vi "Get Function Type.vi"(8 "error in (no error)":errorcluster, 11 "VISA resource name":refnum<visa-resource-name>) -> (0 "error out":errorcluster, 2 "Function Type":i32, 3 "VISA resource name out":refnum<visa-resource-name>)   [LabVIEW 2013, in "Fluke 5XXX Series Multicalibrators.lvlib"]
doc: "This VI returns the present output, measurement, or calibration function.\n\nNote:\n\nThis VI is available only for instrument models 5500A and 5520A."
uses:
  Fluke 5XXX Series Multicalibrators.lvlib
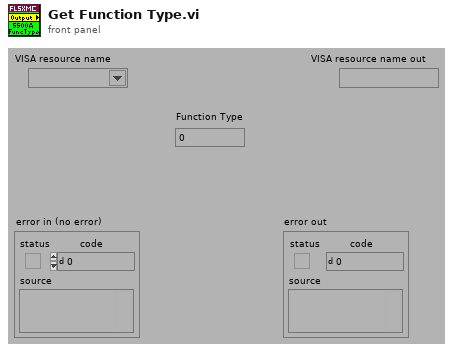
[diagram p1: front panel]
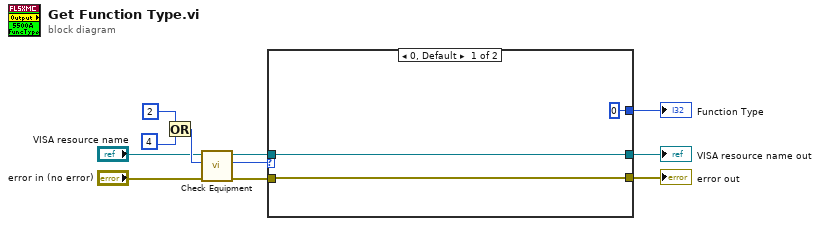
[diagram p0: block diagram]
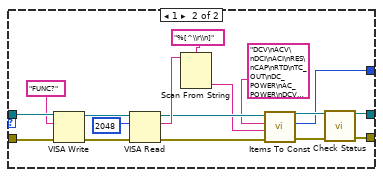
[diagram p2: hidden frame]
diagram:
  n1 = Or(x=2 ("Numeric"), y=4 ("Numeric")) -> (x .or. y?=w8:i32)
  n2 = call "Check Equipment.vi"("error in (no error)"="error in (no error)", "Bit Mask"=w8, "VISA resource name"="VISA resource name") -> ("error out"=w11:errorcluster, "Present?"=w10:u32, "VISA resource name out"=w9:refnum<visa-resource-name>)  [unwired: 6 in]
  n3 = case shown="0, Default" w10 {
    tunnel: [w13 w22] -> w2
    tunnel: w11 -> [w14 w30]
    tunnel: w9 -> [w13 w29]
    tunnel: [w14 w31] -> w3
    tunnel: [0 ("Index") w16] -> w1
    frame 0, Default {
    }
    frame 1 {
      n4 = VISA Write(VISA resource name=w29, write buffer="FUNC?", error in (no error)=w30) -> (VISA resource name out=w26:refnum<visa-resource-name>, error out=w25:errorcluster)  [unwired: 1 out]
      n5 = VISA Read(VISA resource name=w26, byte count=u32 2048 ("byte count (0)"), error in (no error)=w25) -> (VISA resource name out=w19:refnum<visa-resource-name>, read buffer=w23:string, error out=w18:errorcluster)  [unwired: 1 out]
      n6 = Scan From String(format string="%[^\\r\\n]", input string=w23) -> (output 1=w17:string)  [unwired: 3 in, 3 out]
      n7 = call "Items To Const.vi"("error in (no error)"=w18, "String Item"=w17, "Multi-Line String"="DCV\nACV\nDCI\nACI\nRES\nCAP\nRTD\nTC_OUT\nDC_POWER\nAC_POWER\nDCV_DCV\nACV_ACV\nTC_MEAS\nSACV\nSDCV\nMARKER\nLEVSINE\nEDGE\nWAVEGEN\nVIDEO\nPULSE\nMEASZ\nOVERLD", "VISA resource name"=w19) -> ("error out"=w21:errorcluster, "Index"=w16:i32, "VISA resource name out"=w20:refnum<visa-resource-name>)  [unwired: 5 in]
      n8 = call "Check Status.vi"("VISA resource name"=w20, "error in (no error)"=w21) -> ("VISA resource name out"=w22:refnum<visa-resource-name>, "error out"=w31:errorcluster)  [unwired: 12 in]
    }
  }
  "Function Type" <- w1
  "VISA resource name out" <- w2
  "error out" <- w3
